vi "AI Readback All.vi"(7 "Box ID":u8, 8 "error in (no error)":errorcluster, 11 "ENET in":refnum<class "ENET_BS120x.lvclass">) -> (0 "error out":errorcluster, 2 "Voltage":dbl[](array[numeric]), 3 "ENET out":refnum<class "ENET_BS120x.lvclass">)   [LabVIEW 2021, in "BS120x Driver.lvlib" / "ENET_BS120x.lvclass"]
uses:
  ENET_BS120x.lvclass
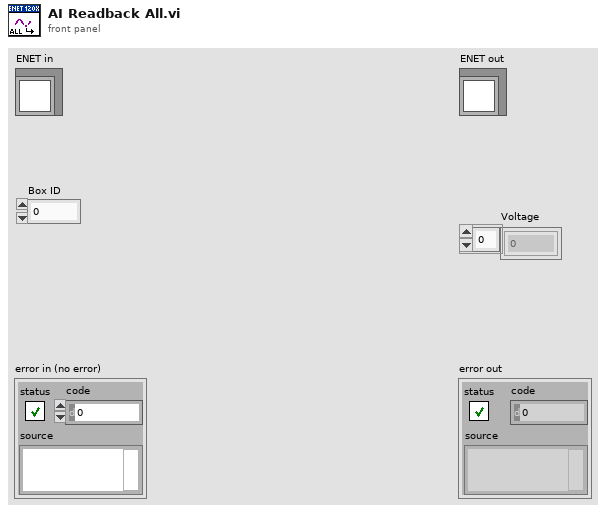
[diagram p1: front panel]
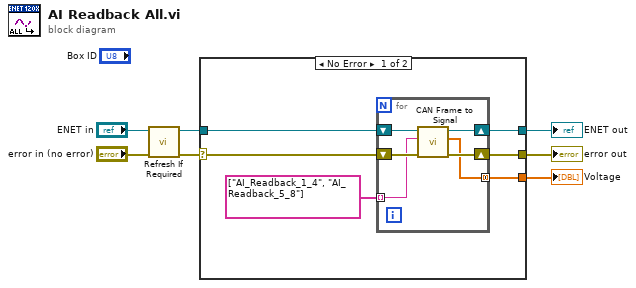
[diagram p0: block diagram]
diagram:
  n1 = call "Refresh If Required.vi"("error in (no error)"="error in (no error)", "Ethernet in"="ENET in") -> ("error out"=w5:errorcluster, "Ethernet out"=w4:refnum<class "ENET_BS120x.lvclass">)  [unwired: 8 in]
  n2 = case shown="No Error" w5 {
    selector: w5 -> [w13 w21]
    tunnel: [w12 w20] -> w2
    tunnel: [w11 w21] -> w3
    tunnel: [w10 _] -> w1
    tunnel: w4 -> [w8 w20]
    frame No Error {
      n3 = for {
        shift-right: [w17] -> w12
        shift-left: w8 -> [w19]
        shift-right: [w16] -> w11
        shift-left: w13 -> [w18]
        tunnel: [w15] -> w10 mode=concatenating
        tunnel: string[] ["AI_Readback_1_4", "AI_Readback_5_8"] -> [w14] mode=indexing
        n4 = call "CAN Frame to Signal.vi"("error in (no error)"=w18, "Frame"=w14, "ENET in"=w19) -> ("error out"=w16:errorcluster, "signal data"=w15:dbl[], "ENET out"=w17:refnum<class "ENET_BS120x.lvclass">)  [unwired: 6 in]
      }
    }
    frame Error {
    }
  }
  "error out" <- w3
  "ENET out" <- w2
  "Voltage" <- w1
